vi "Team Name.vi"(11 "MyTeam":refnum<class "MyTeam.lvclass">) -> (2 "Team Name":string)   [LabVIEW 2020, in "Clones.lvlib" / "MyTeam.lvclass"]
uses:
  MyTeam.lvclass
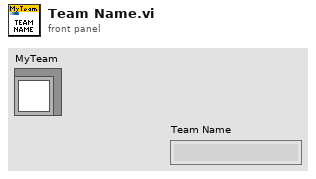
[diagram p1: front panel]
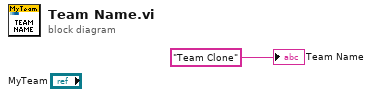
[diagram p0: block diagram]
diagram:
  "Team Name" <- "Team Clone" ("Team Name")
